vi "niRFUtil WFM Detect Edge (real wfm).vi"(0 "Input Waveform":T3 {"y" min=0 max=127 format="%.2f"; "dx" format="%^.2e"; "x0" format="%^.2e"}, 5 "Edge Detection Settings":T1={"Mode"=enum."Sliding Window", "Sliding Window Settings"={"Chunks"=500, "Threshold (dB)"=12.0}, "Threshold Settings"={"Threshold Level (dB)"=-50.0, "Minimum Quiet Time (s)"=5e-05, "Threshold Type"=enum."Absolute"}} {"Threshold Settings"."Minimum Quiet Time (s)" format="%.3p"; "Threshold Settings"."Threshold Level (dB)" format="%.3g"; "Sliding Window Settings"."Threshold (dB)" format="%.3g"}, 7 "Edge Type":T2, 11 "error in (no error)":errorcluster) -> (4 "Output Waveform":T3 {"y" min=0 max=127 format="%.2f"; "dx" format="%^.2e"; "x0" format="%^.2e"}, 6 "Edge Detected?":bool, 8 "Detected Edge Position (s)":dbl format="%^.3e", 15 "error out":errorcluster)   [LabVIEW 2015, in "niRFUtil.lvlib"]
uses:
  niRFUtil.lvlib
  Includes/niRFUtil INC Real Waveform.ctl
  Includes/niRFUtil INC Real Array.ctl
  Includes/niRFUtil INC Edge Type.ctl
  Includes/niRFUtil INC Edge Detection Settings.ctl
  niRFUtil WFM Parse Waveform - Duration (real wfm).vi
  Conversion/niRFUtil CONV 1 Ohm Voltage to dBm (real wfm).vi
  Measurements/niRFUtil MEAS Waveform Statistics (real wfm).vi
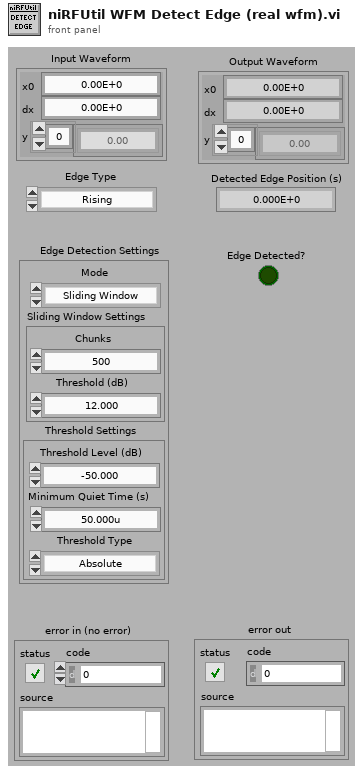
[diagram p1: front panel]
types:
  T1 = typedef "niRFUtil.lvlib/niRFUtil INC Edge Detection Settings.ctl" = cluster{"Mode":enum16{"Sliding Window", "Threshold"}, "Sliding Window Settings":cluster{"Chunks":i32, "Threshold (dB)":dbl}, "Threshold Settings":cluster{"Threshold Level (dB)":dbl, "Minimum Quiet Time (s)":dbl, "Threshold Type":enum16{"Relative", "Absolute"}}}
  T2 = typedef "niRFUtil.lvlib/niRFUtil INC Edge Type.ctl" = enum16{"Rising", "Falling"}
  T3 = typedef "niRFUtil.lvlib/niRFUtil INC Real Waveform.ctl" = cluster{"x0":dbl, "dx":dbl, "y":T4}
  T4 = typedef "niRFUtil.lvlib/niRFUtil INC Real Array.ctl" = sgl[]
  T5 = cluster{"Threshold Level (dB)":dbl, "Minimum Quiet Time (s)":dbl, "Threshold Type":enum16{"Relative", "Absolute"}}
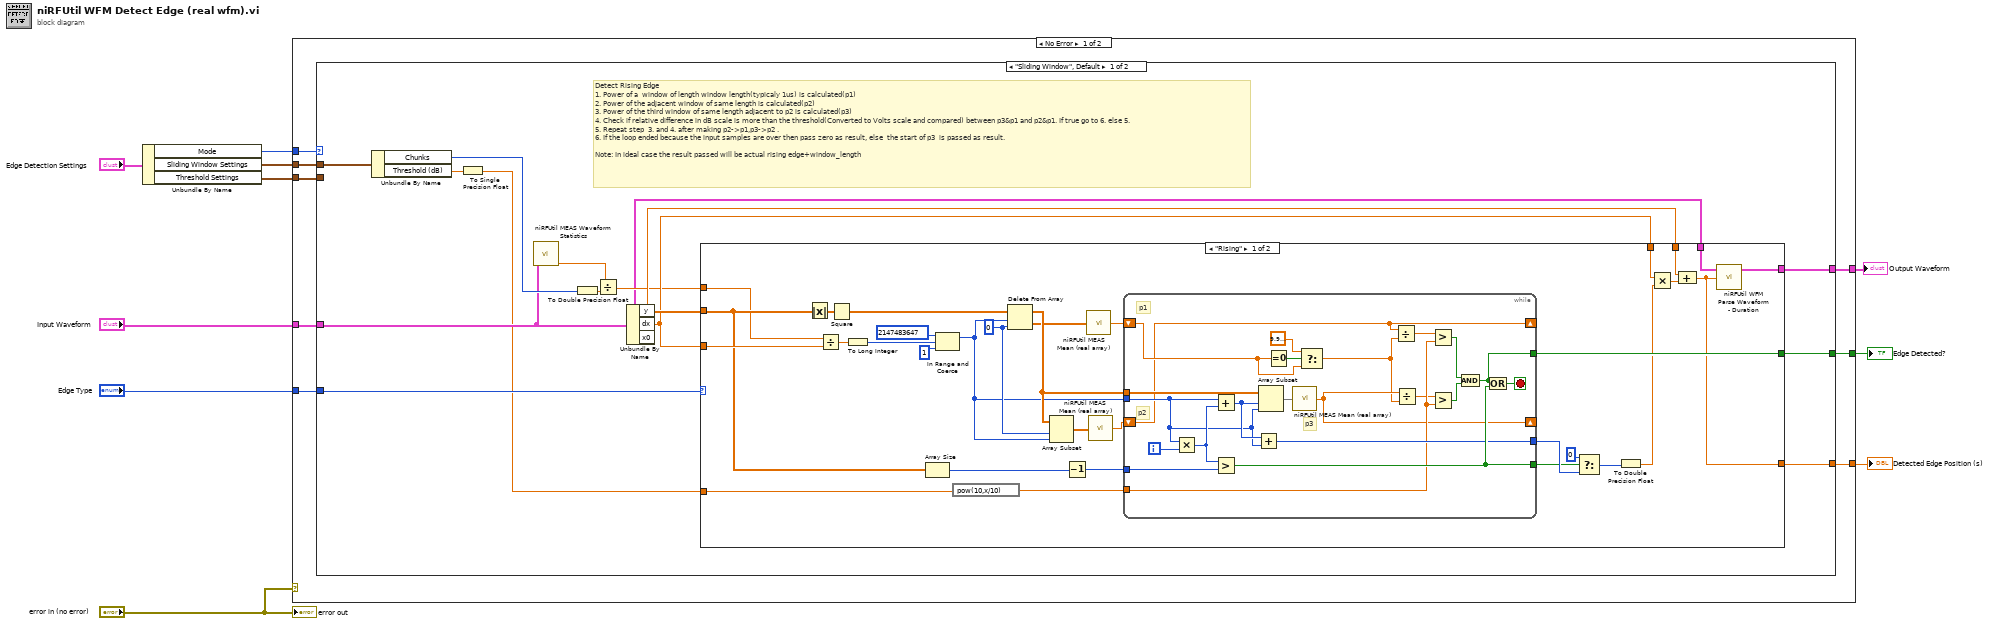
[diagram p0: block diagram]
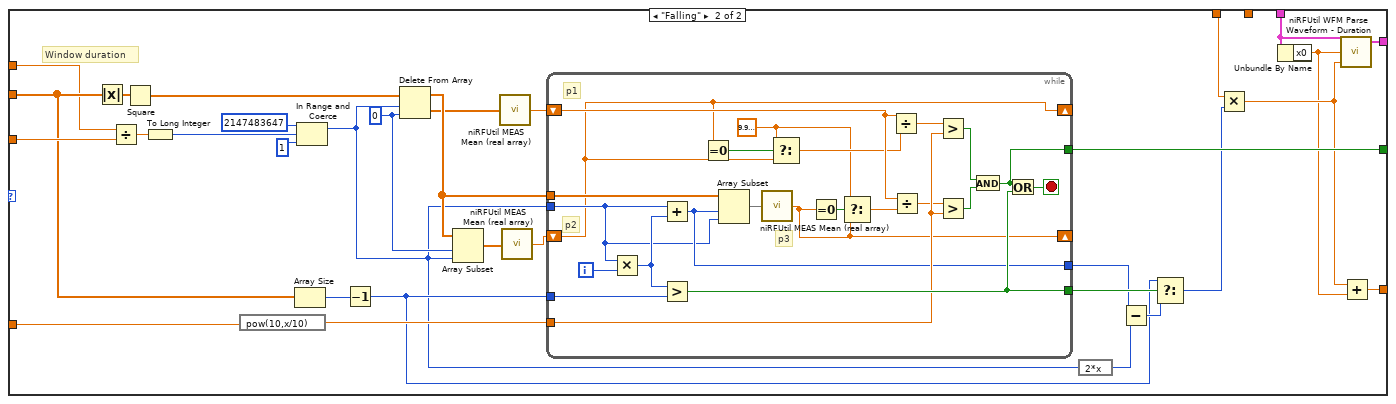
[diagram p2: hidden frame]
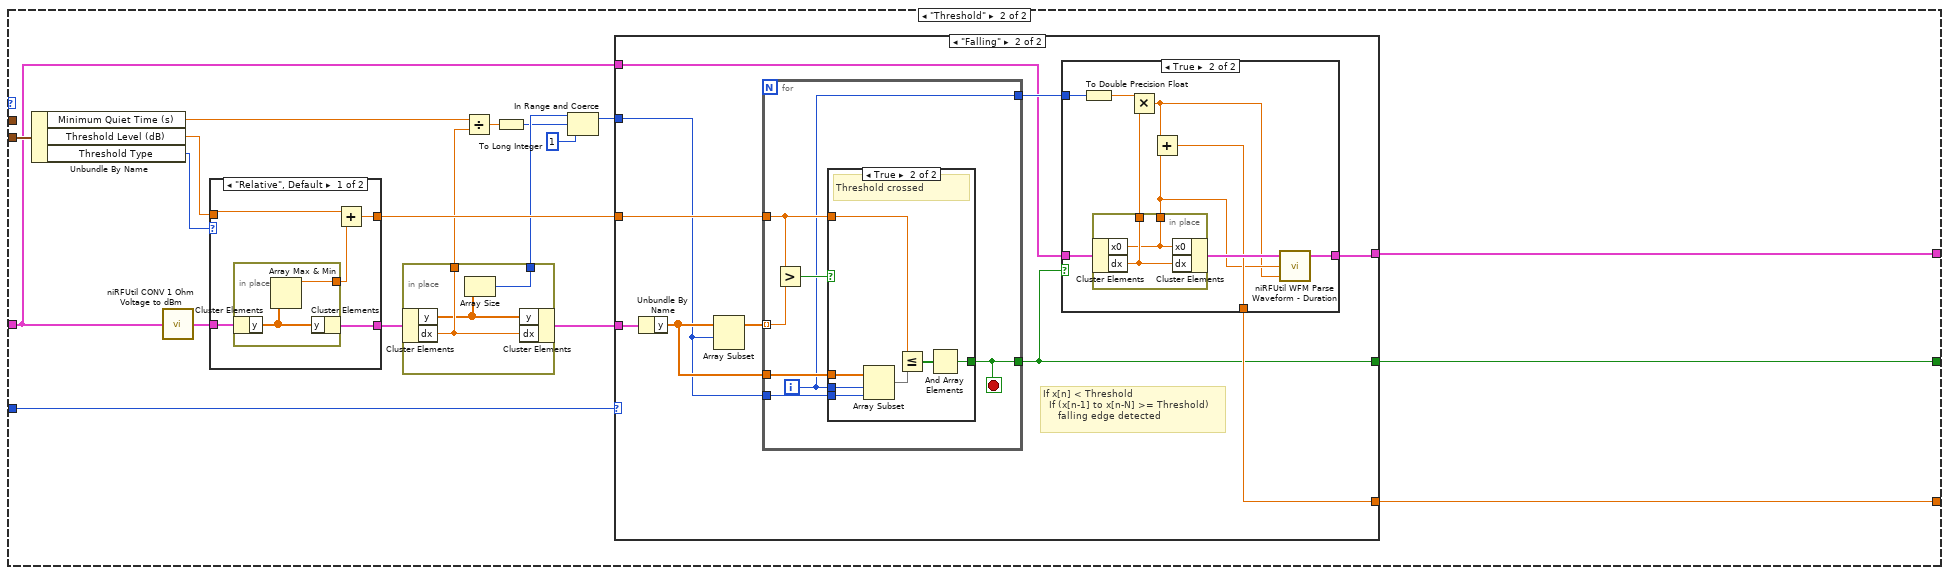
[diagram p3: hidden frame]
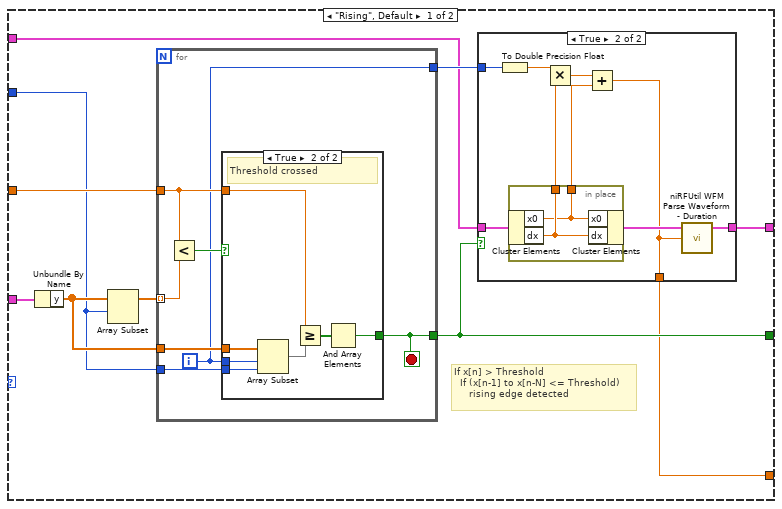
[diagram p4: hidden frame]
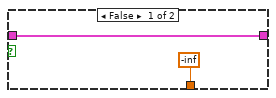
[diagram p5: hidden frame]
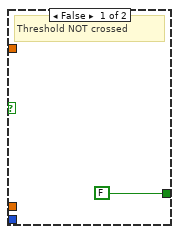
[diagram p6: hidden frame]
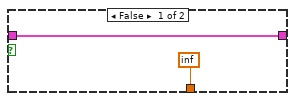
[diagram p7: hidden frame]
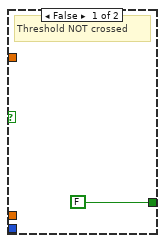
[diagram p8: hidden frame]
diagram:
  n1 = Unbundle By Name("Edge Detection Settings") -> ("Mode"=w3:enum16{"Sliding Window", "Threshold"}, "Sliding Window Settings"=w2:cluster{"Chunks":i32, "Threshold (dB)":dbl}, "Threshold Settings"=w1:T5)
  n2 = case shown="No Error" "error in (no error)" {
    tunnel: [w18 _] -> w10
    tunnel: [w17 _] -> w9
    tunnel: "Edge Type" -> [w16 _]
    tunnel: [w15 _] -> w7
    tunnel: "Input Waveform" -> [w14 _]
    tunnel: w3 -> [w13 _]
    tunnel: w2 -> [w12 _]
    tunnel: w1 -> [w11 _]
    frame No Error {
      n3 = case shown="\"Sliding Window\", Default" w13 {
        tunnel: [w33 w146] -> w18
        tunnel: [w31 w144] -> w17
        tunnel: w16 -> [w30 w157]
        tunnel: [w27 w145] -> w15
        tunnel: w14 -> [w21 w143]
        tunnel: w12 -> [w24 _]
        tunnel: w11 -> [_ w160]
        frame "Sliding Window", Default {
          # "Detect Rising Edge\n1. Power of a  window of length window length(typicaly 1us) is calculated(p1)\n2. Power of the adjacent window of same length is calculated(p2)\n3. Power of the third window of same length adjacent to p2 is calculated(p3)\n4. Check if relative difference in dB scale is more than the threshold(Converted to Volts scale and compared) between p3&p1 and p2&p1. If true go to 6. else 5.\n5. Repeat step  3. and 4. after making p2->p1,p3->p2 .\n6. If the loop ended because the input samples are over then pass zero as result, else  the start of p3  is passed as result.\n\nNote: In ideal case the result passed will be actual rising edge+window_length"
          n4 = Unbundle By Name(w24) -> ("Chunks"=w23:i32, "Threshold (dB)"=w22:dbl)
          n5 = To Single Precision Float(number=w22) -> (single precision float=w19:sgl)
          n6 = call-poly "niRFUtil MEAS Waveform Statistics.vi"("Waveform In"=w21) -> ("Duration"=w26:dbl)  [unwired: 4 in, 3 out]
          n7 = To Double Precision Float(number=w23) -> (double precision float=w20:dbl)
          n8 = Divide(x=w26, y=w20) -> (x/y=w25:dbl)
          n9 = Unbundle By Name(w21) -> ("y"=w32:T4, "dx"=w29:dbl, "x0"=w28:dbl)
          n10 = case shown="\"Rising\"" w30 {
            tunnel: [w39 w94] -> w31
            tunnel: w29 -> [w65 w119]
            tunnel: w32 -> [w64 w118]
            tunnel: [w63 w117] -> w33
            tunnel: w25 -> [w62 w116]
            tunnel: w19 -> [w61 w115]
            tunnel: w29 -> [w44 w101]
            tunnel: w28 -> [w43 _]
            tunnel: w21 -> [w42 w99]
            tunnel: [w41 w102] -> w27
            frame "Rising" {
              w54 = 0 ("index")
              n11 = Absolute Value(x=w64) -> (abs(x)=w49:T4)
              n12 = Divide(x=w62, y=w65) -> (x/y=w59:dbl)
              n13 = Square(x=w49) -> (x^2=w58:T4)
              n14 = To Long Integer(number=w59) -> (32bit integer=w35:i32)
              n15 = Array Size(array=w64) -> (size(s)=w50:i32)
              n16 = In Range and Coerce(upper limit=2147483647, x=w35, lower limit=1) -> (coerced(x)=w34:i32)  [unwired: 1 out]
              n17 = expression code="pow(10,x/10)"(w61) -> (w53:sgl)
              n18 = Delete From Array(array=w58, length=w34, index=w54) -> (deleted portion=w52:T4, array with subset deleted=w55:T4)
              n19 = Array Subset(array=w55, index=w54, length=w34) -> (w56:T4)
              n20 = Decrement(x=w50) -> (x-1=w51:i32)
              n21 = call "niRFUtil MEAS Mean (real array).vi"("Real Array"=w52) -> ("Mean"=w46:sgl)  [unwired: 14 in]
              n22 = call "niRFUtil MEAS Mean (real array).vi"("Real Array"=w56) -> ("Mean"=w57:sgl)  [unwired: 14 in]
              n23 = while {
                tunnel: [w80] -> w48
                tunnel: [w86] -> w47
                tunnel: w51 -> [w85]
                tunnel: w55 -> [w83]
                shift-right: [w67] -> _
                shift-left: w46 -> [w68]
                tunnel: w53 -> [w77]
                tunnel: w34 -> [w69]
                shift-right: [w72] -> _
                shift-left: w57 -> [w67]
                tunnel: [w66] -> w63
                i -> [w76]
                stop <- w87 stop-if-true
                # "p3"
                # "p1"
                # "p2"
                n24 = Multiply(x=w69, y=w76) -> (x*y=w71:i32)
                n25 = Add(x=w69, y=w71) -> (x+y=w75:i32)
                n26 = Greater?(x=w71, y=w85) -> (0:w86:bool)
                n27 = Add(x=w75, y=w69) -> (x+y=w80:i32)
                n28 = Array Subset(array=w83, index=w75, length=w69) -> (w84:T4)
                n29 = Equal To 0?(x=w68) -> (x = 0?=w79:bool)
                n30 = call "niRFUtil MEAS Mean (real array).vi"("Real Array"=w84) -> ("Mean"=w72:sgl)  [unwired: 14 in]
                n31 = Select(t=sgl 1e-06, s=w79, f=w68) -> (s? t:f=w70:sgl)
                n32 = Divide(x=w67, y=w70) -> (x/y=w73:sgl)
                n33 = Divide(x=w72, y=w70) -> (x/y=w74:sgl)
                n34 = Greater?(x=w73, y=w77) -> (0:w82:bool)
                n35 = Greater?(x=w74, y=w77) -> (0:w81:bool)
                n36 = And(x=w82, y=w81) -> (x .and. y?=w66:bool)
                n37 = Or(x=w66, y=w86) -> (x .or. y?=w87:bool)
              }
              n38 = Select(t=0, s=w47, f=w48) -> (s? t:f=w40:i32)
              n39 = To Double Precision Float(number=w40) -> (double precision float=w38:dbl)
              n40 = Multiply(x=w44, y=w38) -> (x*y=w45:dbl)
              n41 = Compound Arithmetic op=ADD(w43, w45) -> (w39:dbl)
              n42 = call-poly "niRFUtil WFM Parse Waveform - Duration.vi"("Start (-Inf)"=w39, "Waveform In"=w42) -> ("Waveform Out"=w41:T3)  [unwired: 3 in]
            }
            frame "Falling" {
              w109 = 0 ("index")
              # "Window duration"
              n43 = Absolute Value(x=w118) -> (abs(x)=w105:T4)
              n44 = Divide(x=w116, y=w119) -> (x/y=w114:dbl)
              n45 = Square(x=w105) -> (x^2=w113:T4)
              n46 = To Long Integer(number=w114) -> (32bit integer=w89:i32)
              n47 = expression code="pow(10,x/10)"(w115) -> (w108:sgl)
              n48 = Array Size(array=w118) -> (size(s)=w106:i32)
              n49 = In Range and Coerce(upper limit=2147483647, x=w89, lower limit=1) -> (coerced(x)=w88:i32)  [unwired: 1 out]
              n50 = Decrement(x=w106) -> (x-1=w95:i32)
              n51 = Delete From Array(array=w113, length=w88, index=w109) -> (deleted portion=w107:T4, array with subset deleted=w110:T4)
              n52 = Array Subset(array=w110, index=w109, length=w88) -> (w111:T4)
              n53 = call "niRFUtil MEAS Mean (real array).vi"("Real Array"=w107) -> ("Mean"=w103:sgl)  [unwired: 14 in]
              n54 = call "niRFUtil MEAS Mean (real array).vi"("Real Array"=w111) -> ("Mean"=w112:sgl)  [unwired: 14 in]
              n55 = while {
                tunnel: [w132] -> w97
                tunnel: [w141] -> w104
                tunnel: w95 -> [w140]
                tunnel: w110 -> [w138]
                shift-right: [w125] -> _
                shift-left: w103 -> [w126]
                tunnel: w108 -> [w134]
                tunnel: w88 -> [w127]
                shift-right: [w122] -> _
                shift-left: w112 -> [w125]
                tunnel: [w129] -> w117
                i -> [w133]
                stop <- w142 stop-if-true
                w120 = sgl 1e-06 ("t")
                # "p3"
                # "p1"
                # "p2"
                n56 = Multiply(x=w127, y=w133) -> (x*y=w128:i32)
                n57 = Add(x=w127, y=w128) -> (x+y=w132:i32)
                n58 = Greater?(x=w128, y=w140) -> (0:w141:bool)
                n59 = Equal To 0?(x=w125) -> (x = 0?=w135:bool)
                n60 = Array Subset(array=w138, index=w132, length=w127) -> (w139:T4)
                n61 = call "niRFUtil MEAS Mean (real array).vi"("Real Array"=w139) -> ("Mean"=w122:sgl)  [unwired: 14 in]
                n62 = Select(t=w120, s=w135, f=w125) -> (s? t:f=w124:sgl)
                n63 = Equal To 0?(x=w122) -> (x = 0?=w123:bool)
                n64 = Select(t=w120, s=w123, f=w122) -> (s? t:f=w121:sgl)
                n65 = Divide(x=w126, y=w124) -> (x/y=w130:sgl)
                n66 = Divide(x=w126, y=w121) -> (x/y=w131:sgl)
                n67 = Greater?(x=w130, y=w134) -> (0:w137:bool)
                n68 = Greater?(x=w131, y=w134) -> (0:w136:bool)
                n69 = And(x=w137, y=w136) -> (x .and. y?=w129:bool)
                n70 = Or(x=w129, y=w141) -> (x .or. y?=w142:bool)
              }
              n71 = expression code="2*x"(w88) -> (w98:i32)
              n72 = Subtract(x=w97, y=w98) -> (x-y=w96:i32)
              n73 = Select(t=w95, s=w104, f=w96) -> (s? t:f=w100:i32)
              n74 = Multiply(x=w101, y=w100) -> (x*y=w93:dbl)
              n75 = Unbundle By Name(w99) -> ("x0"=w92:dbl)
              n76 = call-poly "niRFUtil WFM Parse Waveform - Duration.vi"("Duration (Inf)"=w93, "Start (-Inf)"=w92, "Waveform In"=w99) -> ("Waveform Out"=w102:T3)  [unwired: 2 in]
              n77 = Add(x=w93, y=w92) -> (x+y=w94:dbl)
            }
          }
        }
        frame "Threshold" {
          n78 = Unbundle By Name(w160) -> ("Minimum Quiet Time (s)"=w152:dbl, "Threshold Level (dB)"=w159:dbl, "Threshold Type"=w158:enum16{"Relative", "Absolute"})
          n79 = call-poly "niRFUtil CONV 1 Ohm Voltage to dBm.vi"("Real Waveform (V)"=w143) -> ("Real Waveform (dBm)"=w161:T3)  [unwired: 14 in]
          n80 = case shown="\"Relative\", Default" w158 {
            tunnel: w161 -> [w245 w248]
            tunnel: [w243 w248] -> w155
            tunnel: [w242 w249] -> w156
            tunnel: w159 -> [w241 w249]
            frame "Relative", Default {
              n81 = in-place {
                in-place-border: [w246] -> w244
                n82 = in-place-cluster #1(w245) -> ("y"=w247:T4)
                n83 = Array Max & Min(array=w247) -> (max value=w246:sgl)  [unwired: 3 out]
                n84 = in-place-cluster #1("y"=w247) -> (w243:T3)
              }
              n85 = Add(x=w241, y=w244) -> (x+y=w242:dbl)
            }
            frame "Absolute" {
            }
          }
          n86 = in-place {
            in-place-border: [w164] -> w153
            in-place-border: [w162] -> w149
            n87 = in-place-cluster #2(w155) -> ("y"=w163:T4, "dx"=w164:dbl)
            n88 = Array Size(array=w163) -> (size(s)=w162:i32)
            n89 = in-place-cluster #2("y"=w163, "dx"=w164) -> (w154:T3)
          }
          n90 = Divide(x=w152, y=w153) -> (x/y=w151:dbl)
          n91 = To Long Integer(number=w151) -> (32bit integer=w148:i32)
          n92 = In Range and Coerce(upper limit=w149, x=w148, lower limit=1) -> (coerced(x)=w147:i32)  [unwired: 1 out]
          n93 = case shown="\"Falling\"" w157 {
            tunnel: w154 -> [w170 w207]
            tunnel: w156 -> [w174 w212]
            tunnel: w147 -> [w171 w209]
            tunnel: [w168 w204] -> w146
            tunnel: [w169 w205] -> w145
            tunnel: [w166 w206] -> w144
            tunnel: w143 -> [w165 w203]
            frame "Rising", Default {
              # "If x[n] > Threshold\n  If (x[n-1] to x[n-N] <= Threshold)\n     rising edge detected"
              n94 = Unbundle By Name(w170) -> ("y"=w173:T4)
              n95 = Array Subset(array=w173, index=w171) -> (w172:T4)  [unwired: 1 in]
              n96 = for {
                tunnel: w172 -> [w194] mode=indexing
                tunnel: w174 -> [w190]
                tunnel: w173 -> [w192]
                tunnel: w171 -> [w191]
                tunnel: [w189] -> w168
                tunnel: [w188] -> w167
                i -> [w188]
                stop <- w189 stop-if-true
                n97 = Less?(x=w190, y=w194) -> (x < y?=w193:bool)
                n98 = case shown="True" w193 {
                  tunnel: w192 -> [_ w202]
                  tunnel: w188 -> [_ w201]
                  tunnel: w191 -> [_ w200]
                  tunnel: w190 -> [_ w199]
                  tunnel: [FALSE w196] -> w189
                  frame False {
                    # "Threshold NOT crossed"
                  }
                  frame True {
                    # "Threshold crossed"
                    n99 = Array Subset(array=w202, index=w201, length=w200) -> (w198:T4)
                    n100 = Greater Or Equal?(x=w199, y=w198) -> (x >= y?=w197:bool[])
                    n101 = And Array Elements(Boolean array=w197) -> (logical AND=w196:bool)
                  }
                }
              }
              n102 = case shown="True" w168 {
                tunnel: w165 -> [w176 w184]
                tunnel: [w176 w185] -> w169
                tunnel: w167 -> [_ w182]
                tunnel: [-inf w178] -> w166
                frame False {
                }
                frame True {
                  n103 = To Double Precision Float(number=w182) -> (double precision float=w177:dbl)
                  n104 = in-place {
                    in-place-border: [w187] -> w181
                    in-place-border: [w186] -> w179
                    n105 = in-place-cluster #3(w184) -> ("x0"=w186:dbl, "dx"=w187:dbl)
                    n106 = in-place-cluster #3("x0"=w186, "dx"=w187) -> (w183:T3)
                  }
                  n107 = Multiply(x=w177, y=w181) -> (x*y=w180:dbl)
                  n108 = Add(x=w180, y=w179) -> (x+y=w178:dbl)
                  n109 = call-poly "niRFUtil WFM Parse Waveform - Duration.vi"("Start (-Inf)"=w178, "Waveform In"=w183) -> ("Waveform Out"=w185:T3)  [unwired: 3 in]
                }
              }
            }
            frame "Falling" {
              # "If x[n] < Threshold\n  If (x[n-1] to x[n-N] >= Threshold)\n     falling edge detected"
              n110 = Unbundle By Name(w207) -> ("y"=w211:T4)
              n111 = Array Subset(array=w211, index=w209) -> (w210:T4)  [unwired: 1 in]
              n112 = for {
                tunnel: w210 -> [w232] mode=indexing
                tunnel: w212 -> [w228]
                tunnel: w211 -> [w230]
                tunnel: w209 -> [w229]
                tunnel: [w227] -> w204
                tunnel: [w226] -> w208
                i -> [w226]
                stop <- w227 stop-if-true
                n113 = Greater?(x=w228, y=w232) -> (0:w231:bool)
                n114 = case shown="True" w231 {
                  tunnel: w230 -> [_ w240]
                  tunnel: w226 -> [_ w239]
                  tunnel: w229 -> [_ w238]
                  tunnel: w228 -> [_ w237]
                  tunnel: [FALSE w234] -> w227
                  frame False {
                    # "Threshold NOT crossed"
                  }
                  frame True {
                    # "Threshold crossed"
                    n115 = Array Subset(array=w240, index=w239, length=w238) -> (w236:T4)
                    n116 = Less Or Equal?(x=w237, y=w236) -> (x <= y?=w235:bool[])
                    n117 = And Array Elements(Boolean array=w235) -> (logical AND=w234:bool)
                  }
                }
              }
              n118 = case shown="True" w204 {
                tunnel: w203 -> [w214 w222]
                tunnel: [w214 w223] -> w205
                tunnel: w208 -> [_ w220]
                tunnel: [inf w218] -> w206
                frame False {
                }
                frame True {
                  n119 = To Double Precision Float(number=w220) -> (double precision float=w217:dbl)
                  n120 = in-place {
                    in-place-border: [w225] -> w219
                    in-place-border: [w224] -> w216
                    n121 = in-place-cluster #4(w222) -> ("x0"=w224:dbl, "dx"=w225:dbl)
                    n122 = in-place-cluster #4("x0"=w224, "dx"=w225) -> (w221:T3)
                  }
                  n123 = Multiply(x=w217, y=w219) -> (x*y=w215:dbl)
                  n124 = Add(x=w215, y=w216) -> (x+y=w218:dbl)
                  n125 = call-poly "niRFUtil WFM Parse Waveform - Duration.vi"("Duration (Inf)"=w215, "Start (-Inf)"=w216, "Waveform In"=w221) -> ("Waveform Out"=w223:T3)  [unwired: 2 in]
                }
              }
            }
          }
        }
      }
    }
    frame Error {
    }
  }
  "Detected Edge Position (s)" <- w9
  "Edge Detected?" <- w10
  "Output Waveform" <- w7
  "error out" <- "error in (no error)"
